vi "HandleObservationSync_002.vi"(8 "error in (no error)":errorcluster, 11 "S4GUI in":refnum<class "S4GUI.lvclass">) -> (0 "error out":errorcluster, 3 "S4GUI out":refnum<class "S4GUI.lvclass">)   [LabVIEW 2018, in "S4GUI.lvclass"] (continued)
            }
          }
          n1271 = call "Write AcquisitionB.vi"("error in (no error)"=w3487, "Acquisition.lvclass"=w3489, "S4ACS_GUI in"=w3488) -> ("error out"=w3483:errorcluster, "S4ACS_GUI out"=w3482:refnum<class "S4GUI.lvclass">)  [unwired: 7 in]
          n1272 = call-dynamic "Read AcquisitionC.vi"("error in (no error)"=w3483, "S4ACS_GUI in"=w3482) -> ("error out"=w3440:errorcluster, "Acquisition.lvclass"=w3442:refnum<class "Acquisition.lvclass">, "S4ACS_GUI out"=w3485:refnum<class "S4GUI.lvclass">)  [unwired: 7 in]
          n1273 = call-dynamic "Read enabled.vi"("error in (no error)"=w3440, "Server in"=w3442) -> ("error out"=w3439:errorcluster, "enabled"=w3432:bool, "Server out"=w3441:refnum<class "Acquisition.lvclass">)  [unwired: 7 in]
          n1274 = call "Read connection.vi"("error in (no error)"=w3439, "Server in"=w3441) -> ("error out"=w3469:errorcluster, "connection"=w3452:bool, "Server out"=w3470:refnum<class "Acquisition.lvclass">)  [unwired: 7 in]
          n1275 = And(x=w3452, y=w3432) -> (x .and. y?=w3454:bool)
          n1276 = case shown="True" w3454 {
            tunnel: [w3558 w3567] -> w3486
            tunnel: [w3559 w3566] -> w3484
            tunnel: w3470 -> [w3559 w3564]
            tunnel: w3469 -> [w3558 w3563]
            tunnel: [w3555 u32 0 ("New_State")] -> w3461
            tunnel: w3432 -> [w3554 _]
            frame False {
              n1277 = Select(t=u32 4, s=w3554, f=u32 0) -> (s? t:f=w3555:u32)
            }
            frame True {
              n1278 = call-dynamic "Read Channel.vi"("error in (no error)"=w3563, "Acquisition in"=w3564) -> ("error out"=w3571:errorcluster, "Channel.lvclass"=w3572:refnum<class "Channel.lvclass">, "Acquisition out"=w3565:refnum<class "Acquisition.lvclass">)  [unwired: 7 in]
              n1279 = call-dynamic "Read State Machine.vi"("error in (no error)"=w3571, "Device in"=w3572) -> ("error out"=w3570:errorcluster, "State Machine.lvclass"=w3568:refnum<class "State Machine.lvclass">, "Device out"=w3574:refnum<class "Channel.lvclass">)  [unwired: 7 in]
              n1280 = call "Next State.vi"("error in (no error)"=w3570, "New_State"=50, "State Machine in"=w3568) -> ("error out"=w3562:errorcluster, "State Machine out"=w3561:refnum<class "State Machine.lvclass">)  [unwired: 7 in]
              n1281 = call-dynamic "Write State Machine.vi"("error in (no error)"=w3562, "State Machine.lvclass"=w3561, "Device in"=w3574) -> ("error out"=w3575:errorcluster, "Device out"=w3573:refnum<class "Channel.lvclass">)  [unwired: 7 in]
              n1282 = call-dynamic "Write Channel.vi"("error in (no error)"=w3575, "Channel.lvclass"=w3573, "Acquisition in"=w3565) -> ("error out"=w3567:errorcluster, "Acquisition out"=w3566:refnum<class "Acquisition.lvclass">)  [unwired: 7 in]
            }
          }
          n1283 = call-dynamic "Write AcquisitionC.vi"("error in (no error)"=w3486, "Acquisition.lvclass"=w3484, "S4ACS_GUI in"=w3485) -> ("error out"=w3480:errorcluster, "S4ACS_GUI out"=w3479:refnum<class "S4GUI.lvclass">)  [unwired: 7 in]
          n1284 = call-dynamic "Read AcquisitionD.vi"("error in (no error)"=w3480, "S4ACS_GUI in"=w3479) -> ("error out"=w3436:errorcluster, "Acquisition.lvclass"=w3438:refnum<class "Acquisition.lvclass">, "S4ACS_GUI out"=w3478:refnum<class "S4GUI.lvclass">)  [unwired: 7 in]
          n1285 = call-dynamic "Read enabled.vi"("error in (no error)"=w3436, "Server in"=w3438) -> ("error out"=w3435:errorcluster, "enabled"=w3431:bool, "Server out"=w3437:refnum<class "Acquisition.lvclass">)  [unwired: 7 in]
          n1286 = call "Read connection.vi"("error in (no error)"=w3435, "Server in"=w3437) -> ("error out"=w3467:errorcluster, "connection"=w3451:bool, "Server out"=w3468:refnum<class "Acquisition.lvclass">)  [unwired: 7 in]
          n1287 = And(x=w3451, y=w3431) -> (x .and. y?=w3453:bool)
          n1288 = case shown="True" w3453 {
            tunnel: w3467 -> [w3536 w3553]
            tunnel: [w3536 w3552] -> w3481
            tunnel: w3468 -> [w3537 w3543]
            tunnel: [w3537 w3541] -> w3477
            tunnel: [w3533 u32 0 ("New_State")] -> w3460
            tunnel: w3431 -> [w3532 _]
            frame False {
              n1289 = Select(t=u32 8, s=w3532, f=u32 0) -> (s? t:f=w3533:u32)
            }
            frame True {
              n1290 = call-dynamic "Read Channel.vi"("error in (no error)"=w3553, "Acquisition in"=w3543) -> ("error out"=w3548:errorcluster, "Channel.lvclass"=w3547:refnum<class "Channel.lvclass">, "Acquisition out"=w3542:refnum<class "Acquisition.lvclass">)  [unwired: 7 in]
              n1291 = call-dynamic "Read State Machine.vi"("error in (no error)"=w3548, "Device in"=w3547) -> ("error out"=w3549:errorcluster, "State Machine.lvclass"=w3551:refnum<class "State Machine.lvclass">, "Device out"=w3545:refnum<class "Channel.lvclass">)  [unwired: 7 in]
              n1292 = call "Next State.vi"("error in (no error)"=w3549, "New_State"=50, "State Machine in"=w3551) -> ("error out"=w3539:errorcluster, "State Machine out"=w3540:refnum<class "State Machine.lvclass">)  [unwired: 7 in]
              n1293 = call-dynamic "Write State Machine.vi"("error in (no error)"=w3539, "State Machine.lvclass"=w3540, "Device in"=w3545) -> ("error out"=w3544:errorcluster, "Device out"=w3546:refnum<class "Channel.lvclass">)  [unwired: 7 in]
              n1294 = call-dynamic "Write Channel.vi"("error in (no error)"=w3544, "Channel.lvclass"=w3546, "Acquisition in"=w3542) -> ("error out"=w3552:errorcluster, "Acquisition out"=w3541:refnum<class "Acquisition.lvclass">)  [unwired: 7 in]
            }
          }
          n1295 = call-dynamic "Write AcquisitionD.vi"("error in (no error)"=w3481, "Acquisition.lvclass"=w3477, "S4ACS_GUI in"=w3478) -> ("error out"=w3476:errorcluster, "S4ACS_GUI out"=w3475:refnum<class "S4GUI.lvclass">)  [unwired: 7 in]
          n1296 = Compound Arithmetic op=ADD(w3463, w3462, w3461, w3460) -> (w3464:u32)
          n1297 = case shown="0, Default" w3464 {
            tunnel: w3459 -> [w3501 _ _ _ _ _ _ _ _ _ _ _ _ _ _ _]
            tunnel: [w3500 u32 1 ("Obs_state") u32 1 ("Obs_state") u32 1 ("Obs_state") u32 1 ("Obs_state") u32 1 ("Obs_state") u32 1 ("Obs_state") u32 1 ("Obs_state") u32 1 ("Obs_state") u32 1 ("Obs_state") u32 1 ("Obs_state") u32 1 ("Obs_state") u32 1 ("Obs_state") u32 1 ("Obs_state") u32 1 ("Obs_state") u32 1 ("Obs_state")] -> w3465
            tunnel: ["" ("Error Msg") "ERROR: Lost channel 1 connection... - HandleObservationSync.vi state 323" ("Error Msg") "ERROR: Lost channel 2 connection...- HandleObservationSync.vi state 323" ("Error Msg") "ERROR: Lost channels 1 and 2 connection...- HandleObservationSync.vi state 323" ("Error Msg") "ERROR: Lost channel 3 connection...- HandleObservationSync.vi state 323" ("Error Msg") "ERROR: Lost channels 1 and  3 connection...- HandleObservationSync.vi state 323" ("Error Msg") "ERROR:  Lost channels 2 and  3 connection...- HandleObservationSync.vi state 323" ("Error Msg") "ERROR:  Lost channels 1, 2 and  3 connection...- HandleObservationSync.vi state 323" ("Error Msg") "ERROR: Lost channel 4 connection...- HandleObservationSync.vi state 323" ("Error Msg") "ERROR:  Lost channels 1 and 4 connection...- HandleObservationSync.vi state 323" ("Error Msg") "ERROR:  Lost channels 2 and 4 connection...- HandleObservationSync.vi state 323" ("Error Msg") "ERROR: Lost channels 1, 2 and 4 connection...- HandleObservationSync.vi state 323" ("Error Msg") "ERROR: Lost channels 3 and 4 connection...- HandleObservationSync.vi state 323" ("Error Msg") "ERROR: Lost channels 1, 3 and 4 connection...- HandleObservationSync.vi state 323" ("Error Msg") "ERROR: Lost channels 2, 3 and 4 connection...- HandleObservationSync.vi state 323" ("Error Msg") "ERROR: Lost channels 1, 2, 3 and 4 connection...- HandleObservationSync.vi state 323" ("Error Msg")] -> w3466
            frame 0, Default {
              n1298 = Increment(x=w3501) -> (x+1=w3500:u32)
              n1299 = Tick Count (ms)() -> (millisecond timer value=w3498:u32)
              n1300 = local write "time1"(w3498) -> ()
            }
            frame 1 {
            }
            frame 2 {
            }
            frame 3 {
            }
            frame 4 {
            }
            frame 5 {
            }
            frame 6 {
            }
            frame 7 {
            }
            frame 8 {
            }
            frame 9 {
            }
            frame 10 {
            }
            frame 11 {
            }
            frame 12 {
            }
            frame 13 {
            }
            frame 14 {
            }
            frame 15 {
            }
          }
          n1301 = Bundle By Name(cluster=w3475, "Obs_state"=w3465, "Error Msg"=w3466) -> (w3492:refnum<class "S4GUI.lvclass">)
        }
        frame 324 {
          # "Espera terminar a execução do comando atual \nantes de ir ao proximo passo da Observação."
          n1302 = call-dynamic "Read AcquisitionA.vi"("error in (no error)"=w3670, "S4ACS_GUI in"=w3671) -> ("error out"=w3651:errorcluster, "Acquisition.lvclass"=w3652:refnum<class "Acquisition.lvclass">, "S4ACS_GUI out"=w3673:refnum<class "S4GUI.lvclass">)  [unwired: 7 in]
          n1303 = call "Read connection.vi"("error in (no error)"=w3651, "Server in"=w3652) -> ("error out"=w3650:errorcluster, "connection"=w3649:bool, "Server out"=w3648:refnum<class "Acquisition.lvclass">)  [unwired: 7 in]
          n1304 = case shown="True" w3649 {
            tunnel: w3650 -> [w3770 w3791]
            tunnel: [w3771 w3789] -> w3674
            tunnel: [w3770 w3788] -> w3672
            tunnel: [TRUE w3777] -> w3630
            tunnel: w3648 -> [w3771 w3780]
            tunnel: [FALSE w3772] -> w3628
            frame False {
            }
            frame True {
              n1305 = call-dynamic "Read Channel.vi"("error in (no error)"=w3791, "Acquisition in"=w3780) -> ("error out"=w3774:errorcluster, "Channel.lvclass"=w3776:refnum<class "Channel.lvclass">, "Acquisition out"=w3790:refnum<class "Acquisition.lvclass">)  [unwired: 7 in]
              n1306 = call-dynamic "Read wait_expose.vi"("error in (no error)"=w3774, "Channel in"=w3776) -> ("error out"=w3773:errorcluster, "wait_expose"=w3772:bool, "Channel out"=w3775:refnum<class "Channel.lvclass">)  [unwired: 7 in]
              n1307 = call-dynamic "Read State Machine.vi"("error in (no error)"=w3773, "Device in"=w3775) -> ("error out"=w3782:errorcluster, "State Machine.lvclass"=w3784:refnum<class "State Machine.lvclass">, "Device out"=w3786:refnum<class "Channel.lvclass">)  [unwired: 7 in]
              n1308 = call-dynamic "Read State.vi"("error in (no error)"=w3782, "State Machine in"=w3784) -> ("error out"=w3781:errorcluster, "State"=w3778:i32, "State Machine out"=w3783:refnum<class "State Machine.lvclass">)  [unwired: 7 in]
              n1309 = Greater?(x=w3778, y=53 ("x")) -> (0:w3777:bool)
              n1310 = call-dynamic "Write State Machine.vi"("error in (no error)"=w3781, "State Machine.lvclass"=w3783, "Device in"=w3786) -> ("error out"=w3785:errorcluster, "Device out"=w3787:refnum<class "Channel.lvclass">)  [unwired: 7 in]
              n1311 = call-dynamic "Write Channel.vi"("error in (no error)"=w3785, "Channel.lvclass"=w3787, "Acquisition in"=w3790) -> ("error out"=w3788:errorcluster, "Acquisition out"=w3789:refnum<class "Acquisition.lvclass">)  [unwired: 7 in]
            }
          }
          n1312 = call-dynamic "Write AcquisitionA.vi"("error in (no error)"=w3672, "Acquisition.lvclass"=w3674, "S4ACS_GUI in"=w3673) -> ("error out"=w3667:errorcluster, "S4ACS_GUI out"=w3666:refnum<class "S4GUI.lvclass">)  [unwired: 7 in]
          n1313 = call "Read AcquisitionB.vi"("error in (no error)"=w3667, "S4ACS_GUI in"=w3666) -> ("error out"=w3643:errorcluster, "Acquisition.lvclass"=w3647:refnum<class "Acquisition.lvclass">, "S4ACS_GUI out"=w3668:refnum<class "S4GUI.lvclass">)  [unwired: 7 in]
          n1314 = call "Read connection.vi"("error in (no error)"=w3643, "Server in"=w3647) -> ("error out"=w3644:errorcluster, "connection"=w3645:bool, "Server out"=w3646:refnum<class "Acquisition.lvclass">)  [unwired: 7 in]
          n1315 = case shown="True" w3645 {
            tunnel: w3644 -> [w3746 w3759]
            tunnel: w3646 -> [w3747 w3758]
            tunnel: [TRUE w3753] -> w3632
            tunnel: [w3746 w3757] -> w3665
            tunnel: [w3747 w3756] -> w3664
            tunnel: [FALSE w3748] -> w3627
            frame False {
            }
            frame True {
              n1316 = call-dynamic "Read Channel.vi"("error in (no error)"=w3759, "Acquisition in"=w3758) -> ("error out"=w3750:errorcluster, "Channel.lvclass"=w3752:refnum<class "Channel.lvclass">, "Acquisition out"=w3760:refnum<class "Acquisition.lvclass">)  [unwired: 7 in]
              n1317 = call-dynamic "Read wait_expose.vi"("error in (no error)"=w3750, "Channel in"=w3752) -> ("error out"=w3749:errorcluster, "wait_expose"=w3748:bool, "Channel out"=w3751:refnum<class "Channel.lvclass">)  [unwired: 7 in]
              n1318 = call-dynamic "Read State Machine.vi"("error in (no error)"=w3749, "Device in"=w3751) -> ("error out"=w3766:errorcluster, "State Machine.lvclass"=w3764:refnum<class "State Machine.lvclass">, "Device out"=w3762:refnum<class "Channel.lvclass">)  [unwired: 7 in]
              n1319 = call-dynamic "Read State.vi"("error in (no error)"=w3766, "State Machine in"=w3764) -> ("error out"=w3767:errorcluster, "State"=w3755:i32, "State Machine out"=w3765:refnum<class "State Machine.lvclass">)  [unwired: 7 in]
              n1320 = Greater?(x=w3755, y=53 ("x")) -> (0:w3753:bool)
              n1321 = call-dynamic "Write State Machine.vi"("error in (no error)"=w3767, "State Machine.lvclass"=w3765, "Device in"=w3762) -> ("error out"=w3763:errorcluster, "Device out"=w3761:refnum<class "Channel.lvclass">)  [unwired: 7 in]
              n1322 = call-dynamic "Write Channel.vi"("error in (no error)"=w3763, "Channel.lvclass"=w3761, "Acquisition in"=w3760) -> ("error out"=w3757:errorcluster, "Acquisition out"=w3756:refnum<class "Acquisition.lvclass">)  [unwired: 7 in]
            }
          }
          n1323 = call "Write AcquisitionB.vi"("error in (no error)"=w3665, "Acquisition.lvclass"=w3664, "S4ACS_GUI in"=w3668) -> ("error out"=w3657:errorcluster, "S4ACS_GUI out"=w3656:refnum<class "S4GUI.lvclass">)  [unwired: 7 in]
          n1324 = call-dynamic "Read AcquisitionC.vi"("error in (no error)"=w3657, "S4ACS_GUI in"=w3656) -> ("error out"=w3639:errorcluster, "Acquisition.lvclass"=w3642:refnum<class "Acquisition.lvclass">, "S4ACS_GUI out"=w3659:refnum<class "S4GUI.lvclass">)  [unwired: 7 in]
          n1325 = call "Read connection.vi"("error in (no error)"=w3639, "Server in"=w3642) -> ("error out"=w3638:errorcluster, "connection"=w3640:bool, "Server out"=w3641:refnum<class "Acquisition.lvclass">)  [unwired: 7 in]
          n1326 = case shown="True" w3640 {
            tunnel: [w3722 w3736] -> w3660
            tunnel: [w3723 w3735] -> w3658
            tunnel: w3638 -> [w3722 w3732]
            tunnel: w3641 -> [w3723 w3733]
            tunnel: [TRUE w3729] -> w3631
            tunnel: [FALSE w3724] -> w3626
            frame False {
            }
            frame True {
              n1327 = call-dynamic "Read Channel.vi"("error in (no error)"=w3732, "Acquisition in"=w3733) -> ("error out"=w3726:errorcluster, "Channel.lvclass"=w3728:refnum<class "Channel.lvclass">, "Acquisition out"=w3734:refnum<class "Acquisition.lvclass">)  [unwired: 7 in]
              n1328 = call-dynamic "Read wait_expose.vi"("error in (no error)"=w3726, "Channel in"=w3728) -> ("error out"=w3725:errorcluster, "wait_expose"=w3724:bool, "Channel out"=w3727:refnum<class "Channel.lvclass">)  [unwired: 7 in]
              n1329 = call-dynamic "Read State Machine.vi"("error in (no error)"=w3725, "Device in"=w3727) -> ("error out"=w3742:errorcluster, "State Machine.lvclass"=w3740:refnum<class "State Machine.lvclass">, "Device out"=w3738:refnum<class "Channel.lvclass">)  [unwired: 7 in]
              n1330 = call-dynamic "Read State.vi"("error in (no error)"=w3742, "State Machine in"=w3740) -> ("error out"=w3743:errorcluster, "State"=w3730:i32, "State Machine out"=w3741:refnum<class "State Machine.lvclass">)  [unwired: 7 in]
              n1331 = Greater?(x=w3730, y=53 ("x")) -> (0:w3729:bool)
              n1332 = call-dynamic "Write State Machine.vi"("error in (no error)"=w3743, "State Machine.lvclass"=w3741, "Device in"=w3738) -> ("error out"=w3739:errorcluster, "Device out"=w3737:refnum<class "Channel.lvclass">)  [unwired: 7 in]
              n1333 = call-dynamic "Write Channel.vi"("error in (no error)"=w3739, "Channel.lvclass"=w3737, "Acquisition in"=w3734) -> ("error out"=w3736:errorcluster, "Acquisition out"=w3735:refnum<class "Acquisition.lvclass">)  [unwired: 7 in]
            }
          }
          n1334 = call-dynamic "Write AcquisitionC.vi"("error in (no error)"=w3660, "Acquisition.lvclass"=w3658, "S4ACS_GUI in"=w3659) -> ("error out"=w3654:errorcluster, "S4ACS_GUI out"=w3655:refnum<class "S4GUI.lvclass">)  [unwired: 7 in]
          n1335 = call-dynamic "Read AcquisitionD.vi"("error in (no error)"=w3654, "S4ACS_GUI in"=w3655) -> ("error out"=w3634:errorcluster, "Acquisition.lvclass"=w3637:refnum<class "Acquisition.lvclass">, "S4ACS_GUI out"=w3661:refnum<class "S4GUI.lvclass">)  [unwired: 7 in]
          n1336 = call "Read connection.vi"("error in (no error)"=w3634, "Server in"=w3637) -> ("error out"=w3633:errorcluster, "connection"=w3635:bool, "Server out"=w3636:refnum<class "Acquisition.lvclass">)  [unwired: 7 in]
          n1337 = case shown="True" w3635 {
            tunnel: [w3699 w3719] -> w3663
            tunnel: [w3698 w3718] -> w3662
            tunnel: w3636 -> [w3699 w3717]
            tunnel: w3633 -> [w3698 w3716]
            tunnel: [TRUE w3705] -> w3629
            tunnel: [FALSE w3700] -> w3625
            frame False {
            }
            frame True {
              n1338 = call-dynamic "Read Channel.vi"("error in (no error)"=w3716, "Acquisition in"=w3717) -> ("error out"=w3702:errorcluster, "Channel.lvclass"=w3704:refnum<class "Channel.lvclass">, "Acquisition out"=w3715:refnum<class "Acquisition.lvclass">)  [unwired: 7 in]
              n1339 = call-dynamic "Read wait_expose.vi"("error in (no error)"=w3702, "Channel in"=w3704) -> ("error out"=w3701:errorcluster, "wait_expose"=w3700:bool, "Channel out"=w3703:refnum<class "Channel.lvclass">)  [unwired: 7 in]
              n1340 = call-dynamic "Read State Machine.vi"("error in (no error)"=w3701, "Device in"=w3703) -> ("error out"=w3709:errorcluster, "State Machine.lvclass"=w3711:refnum<class "State Machine.lvclass">, "Device out"=w3713:refnum<class "Channel.lvclass">)  [unwired: 7 in]
              n1341 = call-dynamic "Read State.vi"("error in (no error)"=w3709, "State Machine in"=w3711) -> ("error out"=w3708:errorcluster, "State"=w3706:i32, "State Machine out"=w3710:refnum<class "State Machine.lvclass">)  [unwired: 7 in]
              n1342 = Greater?(x=w3706, y=53 ("x")) -> (0:w3705:bool)
              n1343 = call-dynamic "Write State Machine.vi"("error in (no error)"=w3708, "State Machine.lvclass"=w3710, "Device in"=w3713) -> ("error out"=w3712:errorcluster, "Device out"=w3714:refnum<class "Channel.lvclass">)  [unwired: 7 in]
              n1344 = call-dynamic "Write Channel.vi"("error in (no error)"=w3712, "Channel.lvclass"=w3714, "Acquisition in"=w3715) -> ("error out"=w3718:errorcluster, "Acquisition out"=w3719:refnum<class "Acquisition.lvclass">)  [unwired: 7 in]
            }
          }
          n1345 = call-dynamic "Write AcquisitionD.vi"("error in (no error)"=w3662, "Acquisition.lvclass"=w3663, "S4ACS_GUI in"=w3661) -> ("error out"=w3653:errorcluster, "S4ACS_GUI out"=w3624:refnum<class "S4GUI.lvclass">)  [unwired: 7 in]
          n1346 = Compound Arithmetic op=AND(w3630, w3632, w3631, w3629) -> (w3623:bool)
          n1347 = Compound Arithmetic op=OR(w3628, w3627, w3626, w3625) -> (w3621:bool)
          n1348 = case shown="True" w3623 {
            tunnel: w3624 -> [w3676 w3695]
            tunnel: [w3682 w3694] -> w3620
            tunnel: w3622 -> [_ w3693]
            tunnel: w3621 -> [_ w3689]
            frame False {
              # "Aguardando iniciar exposição por 5s"
              n1349 = Tick Count (ms)() -> (millisecond timer value=w3681:u32)
              n1350 = local read "time1"() -> (w3675:u32)
              n1351 = Subtract(x=w3681, y=w3675) -> (x-y=w3678:u32)
              n1352 = To Double Precision Float(number=w3678) -> (double precision float=w3680:dbl)
              n1353 = Less?(x=5000.0 ("y"), y=w3680) -> (x < y?=w3679:bool)
              n1354 = case shown="True" w3679 {
                tunnel: w3676 -> [w3683 w3687]
                tunnel: [w3683 w3686] -> w3682
                frame False {
                }
                frame True {
                  n1355 = Bundle By Name(cluster=w3687, "Obs_state"=u32 1, "Error Msg"="ERROR: Acquisition Timeout. HandleObservationSync.vi - state 324.") -> (w3686:refnum<class "S4GUI.lvclass">)
                }
              }
            }
            frame True {
              # "327: Verifica incremento de ciclo."
              # "Iniciou aquisição..."
              n1356 = Increment(x=w3693) -> (x+1=w3690:u32)
              n1357 = Select(t=u32 327, s=w3689, f=w3690) -> (s? t:f=w3688:u32)
              n1358 = Tick Count (ms)() -> (millisecond timer value=w3692:u32)
              n1359 = Bundle By Name(cluster=w3695, "Obs_state"=w3688) -> (w3694:refnum<class "S4GUI.lvclass">)
              n1360 = local write "time307"(w3692) -> ()
            }
          }
          n1361 = Bundle By Name(cluster=w3620, "mode EXPOSE"=w3621) -> (w3669:refnum<class "S4GUI.lvclass">)
        }
        frame 325 {
          n1362 = Unbundle By Name(w3801) -> ("mode EXPOSE"=w3800:bool)
          n1363 = case shown="True" w3800 {
            tunnel: w3801 -> [w3854 w3921]
            tunnel: w3806 -> [w3853 w3920]
            tunnel: [w3852 w3918] -> w3805
            tunnel: [w3851 w3919] -> w3804
            tunnel: [w3850 w3917] -> w3794
            tunnel: w3802 -> [w3842 w3917]
            tunnel: [w3841 w3882] -> w3799
            tunnel: [w3841 w3881] -> w3798
            tunnel: [w3841 w3880] -> w3797
            tunnel: [w3841 w3879] -> w3796
            frame False {
              w3841 = 0
              n1364 = call-dynamic "Read Sync Box.lvclass.vi"("error in (no error)"=w3853, "SPARC4_AC in"=w3854) -> ("error out"=w3847:errorcluster, "Sync Box.lvclass"=w3849:refnum<class "Sync Box.lvclass">, "SPARC4_AC out"=w3844:refnum<class "S4GUI.lvclass">)  [unwired: 7 in]
              n1365 = call "Read connection.vi"("error in (no error)"=w3847, "Server in"=w3849) -> ("error out"=w3846:errorcluster, "connection"=w3845:bool, "Server out"=w3848:refnum<class "Sync Box.lvclass">)  [unwired: 7 in]
              n1366 = case shown="True" w3845 {
                tunnel: w3846 -> [w3860 w3878]
                tunnel: [w3861 w3876] -> w3856
                tunnel: [w3860 w3863] -> w3855
                tunnel: w3842 -> [w3857 w3862]
                tunnel: [w3859 w3862] -> w3850
                tunnel: w3848 -> [w3861 w3867]
                tunnel: w3844 -> [w3858 w3864]
                tunnel: [w3858 w3864] -> w3843
                frame False {
                  n1367 = Increment(x=w3857) -> (x+1=w3859:u32)
                }
                frame True {
                  # "Envia comando FIRE para o SyncBox"
                  n1368 = call-dynamic "Read Trigger.lvclass.vi"("error in (no error)"=w3878, "Sync Box in"=w3867) -> ("error out"=w3872:errorcluster, "Trigger.lvclass"=w3871:refnum<class "Trigger.lvclass">, "Sync Box out"=w3877:refnum<class "Sync Box.lvclass">)  [unwired: 7 in]
                  n1369 = call-dynamic "Read State Machine.vi"("error in (no error)"=w3872, "Device in"=w3871) -> ("error out"=w3873:errorcluster, "State Machine.lvclass"=w3875:refnum<class "State Machine.lvclass">, "Device out"=w3869:refnum<class "Trigger.lvclass">)  [unwired: 7 in]
                  n1370 = call "Next State.vi"("error in (no error)"=w3873, "New_State"=40, "State Machine in"=w3875) -> ("error out"=w3865:errorcluster, "State Machine out"=w3866:refnum<class "State Machine.lvclass">)  [unwired: 7 in]
                  n1371 = call-dynamic "Write State Machine.vi"("error in (no error)"=w3865, "State Machine.lvclass"=w3866, "Device in"=w3869) -> ("error out"=w3868:errorcluster, "Device out"=w3870:refnum<class "Trigger.lvclass">)  [unwired: 7 in]
                  n1372 = call-dynamic "Write Trigger.lvclass.vi"("error in (no error)"=w3868, "Trigger.lvclass"=w3870, "Sync Box in"=w3877) -> ("error out"=w3863:errorcluster, "Sync Box out"=w3876:refnum<class "Sync Box.lvclass">)  [unwired: 7 in]
                }
              }
              n1373 = call-dynamic "Write Sync Box.lvclass.vi"("error in (no error)"=w3855, "Sync Box.lvclass"=w3856, "SPARC4_AC in"=w3843) -> ("error out"=w3852:errorcluster, "SPARC4_AC out"=w3851:refnum<class "S4GUI.lvclass">)  [unwired: 7 in]
            }
            frame True {
              # "Envia comando EXPOSE para os canais ativos"
              n1374 = call-dynamic "Read AcquisitionA.vi"("error in (no error)"=w3920, "S4ACS_GUI in"=w3921) -> ("error out"=w3914:errorcluster, "Acquisition.lvclass"=w3916:refnum<class "Acquisition.lvclass">, "S4ACS_GUI out"=w3940:refnum<class "S4GUI.lvclass">)  [unwired: 7 in]
              n1375 = call-dynamic "Read enabled.vi"("error in (no error)"=w3914, "Server in"=w3916) -> ("error out"=w3913:errorcluster, "enabled"=w3886:bool, "Server out"=w3915:refnum<class "Acquisition.lvclass">)  [unwired: 7 in]
              n1376 = call "Read connection.vi"("error in (no error)"=w3913, "Server in"=w3915) -> ("error out"=w3922:errorcluster, "connection"=w3911:bool, "Server out"=w3923:refnum<class "Acquisition.lvclass">)  [unwired: 7 in]
              n1377 = And(x=w3911, y=w3886) -> (x .and. y?=w3912:bool)
              n1378 = case shown="True" w3912 {
                tunnel: w3923 -> [w4013 w4029]
                tunnel: w3922 -> [w4012 w4028]
                tunnel: [w4013 w4026] -> w3941
                tunnel: [w4012 w4025] -> w3939
                tunnel: [w4008 0] -> w3882
                tunnel: w3886 -> [w4009 _]
                frame False {
                  n1379 = Select(t=1, s=w4009, f=0) -> (s? t:f=w4008:i32)
                }
                frame True {
                  n1380 = call-dynamic "Read Channel.vi"("error in (no error)"=w4028, "Acquisition in"=w4029) -> ("error out"=w4021:errorcluster, "Channel.lvclass"=w4020:refnum<class "Channel.lvclass">, "Acquisition out"=w4027:refnum<class "Acquisition.lvclass">)  [unwired: 7 in]
                  n1381 = call-dynamic "Read State Machine.vi"("error in (no error)"=w4021, "Device in"=w4020) -> ("error out"=w4022:errorcluster, "State Machine.lvclass"=w4024:refnum<class "State Machine.lvclass">, "Device out"=w4018:refnum<class "Channel.lvclass">)  [unwired: 7 in]
                  n1382 = call "Next State.vi"("error in (no error)"=w4022, "New_State"=50, "State Machine in"=w4024) -> ("error out"=w4015:errorcluster, "State Machine out"=w4016:refnum<class "State Machine.lvclass">)  [unwired: 7 in]
                  n1383 = call-dynamic "Write State Machine.vi"("error in (no error)"=w4015, "State Machine.lvclass"=w4016, "Device in"=w4018) -> ("error out"=w4017:errorcluster, "Device out"=w4019:refnum<class "Channel.lvclass">)  [unwired: 7 in]
                  n1384 = call-dynamic "Write Channel.vi"("error in (no error)"=w4017, "Channel.lvclass"=w4019, "Acquisition in"=w4027) -> ("error out"=w4025:errorcluster, "Acquisition out"=w4026:refnum<class "Acquisition.lvclass">)  [unwired: 7 in]
                }
              }
              n1385 = call-dynamic "Write AcquisitionA.vi"("error in (no error)"=w3939, "Acquisition.lvclass"=w3941, "S4ACS_GUI in"=w3940) -> ("error out"=w3937:errorcluster, "S4ACS_GUI out"=w3938:refnum<class "S4GUI.lvclass">)  [unwired: 7 in]
              n1386 = call "Read AcquisitionB.vi"("error in (no error)"=w3937, "S4ACS_GUI in"=w3938) -> ("error out"=w3905:errorcluster, "Acquisition.lvclass"=w3907:refnum<class "Acquisition.lvclass">, "S4ACS_GUI out"=w3935:refnum<class "S4GUI.lvclass">)  [unwired: 7 in]
              n1387 = call-dynamic "Read enabled.vi"("error in (no error)"=w3905, "Server in"=w3907) -> ("error out"=w3909:errorcluster, "enabled"=w3885:bool, "Server out"=w3910:refnum<class "Acquisition.lvclass">)  [unwired: 7 in]
              n1388 = call "Read connection.vi"("error in (no error)"=w3909, "Server in"=w3910) -> ("error out"=w3904:errorcluster, "connection"=w3908:bool, "Server out"=w3906:refnum<class "Acquisition.lvclass">)  [unwired: 7 in]
              n1389 = And(x=w3908, y=w3885) -> (x .and. y?=w3903:bool)
              n1390 = case shown="False" w3903 {
                tunnel: w3906 -> [w3991 w4007]
                tunnel: w3904 -> [w3990 w4006]
                tunnel: [w3991 w4004] -> w3936
                tunnel: [w3990 w4003] -> w3934
                tunnel: [w3987 0] -> w3881
                tunnel: w3885 -> [w3986 _]
                frame False {
                  n1391 = Select(t=2, s=w3986, f=0) -> (s? t:f=w3987:i32)
                }
                frame True {
                  n1392 = call-dynamic "Read Channel.vi"("error in (no error)"=w4006, "Acquisition in"=w4007) -> ("error out"=w3999:errorcluster, "Channel.lvclass"=w3998:refnum<class "Channel.lvclass">, "Acquisition out"=w4005:refnum<class "Acquisition.lvclass">)  [unwired: 7 in]
                  n1393 = call-dynamic "Read State Machine.vi"("error in (no error)"=w3999, "Device in"=w3998) -> ("error out"=w4000:errorcluster, "State Machine.lvclass"=w4002:refnum<class "State Machine.lvclass">, "Device out"=w3996:refnum<class "Channel.lvclass">)  [unwired: 7 in]
                  n1394 = call "Next State.vi"("error in (no error)"=w4000, "New_State"=50, "State Machine in"=w4002) -> ("error out"=w3993:errorcluster, "State Machine out"=w3994:refnum<class "State Machine.lvclass">)  [unwired: 7 in]
                  n1395 = call-dynamic "Write State Machine.vi"("error in (no error)"=w3993, "State Machine.lvclass"=w3994, "Device in"=w3996) -> ("error out"=w3995:errorcluster, "Device out"=w3997:refnum<class "Channel.lvclass">)  [unwired: 7 in]
                  n1396 = call-dynamic "Write Channel.vi"("error in (no error)"=w3995, "Channel.lvclass"=w3997, "Acquisition in"=w4005) -> ("error out"=w4003:errorcluster, "Acquisition out"=w4004:refnum<class "Acquisition.lvclass">)  [unwired: 7 in]
                }
              }
              n1397 = call "Write AcquisitionB.vi"("error in (no error)"=w3934, "Acquisition.lvclass"=w3936, "S4ACS_GUI in"=w3935) -> ("error out"=w3930:errorcluster, "S4ACS_GUI out"=w3929:refnum<class "S4GUI.lvclass">)  [unwired: 7 in]
              n1398 = call-dynamic "Read AcquisitionC.vi"("error in (no error)"=w3930, "S4ACS_GUI in"=w3929) -> ("error out"=w3896:errorcluster, "Acquisition.lvclass"=w3897:refnum<class "Acquisition.lvclass">, "S4ACS_GUI out"=w3932:refnum<class "S4GUI.lvclass">)  [unwired: 7 in]
              n1399 = call-dynamic "Read enabled.vi"("error in (no error)"=w3896, "Server in"=w3897) -> ("error out"=w3901:errorcluster, "enabled"=w3884:bool, "Server out"=w3902:refnum<class "Acquisition.lvclass">)  [unwired: 7 in]
              n1400 = call "Read connection.vi"("error in (no error)"=w3901, "Server in"=w3902) -> ("error out"=w3898:errorcluster, "connection"=w3900:bool, "Server out"=w3899:refnum<class "Acquisition.lvclass">)  [unwired: 7 in]
              n1401 = And(x=w3900, y=w3884) -> (x .and. y?=w3895:bool)
              n1402 = case shown="False" w3895 {
                tunnel: [w3968 w3977] -> w3933
                tunnel: [w3969 w3976] -> w3931
                tunnel: w3899 -> [w3969 w3974]
                tunnel: w3898 -> [w3968 w3973]
                tunnel: [w3964 0] -> w3880
                tunnel: w3884 -> [w3965 _]
                frame False {
                  n1403 = Select(t=4, s=w3965, f=0) -> (s? t:f=w3964:i32)
                }
                frame True {
                  n1404 = call-dynamic "Read Channel.vi"("error in (no error)"=w3973, "Acquisition in"=w3974) -> ("error out"=w3981:errorcluster, "Channel.lvclass"=w3982:refnum<class "Channel.lvclass">, "Acquisition out"=w3975:refnum<class "Acquisition.lvclass">)  [unwired: 7 in]
                  n1405 = call-dynamic "Read State Machine.vi"("error in (no error)"=w3981, "Device in"=w3982) -> ("error out"=w3980:errorcluster, "State Machine.lvclass"=w3978:refnum<class "State Machine.lvclass">, "Device out"=w3984:refnum<class "Channel.lvclass">)  [unwired: 7 in]
                  n1406 = call "Next State.vi"("error in (no error)"=w3980, "New_State"=50, "State Machine in"=w3978) -> ("error out"=w3972:errorcluster, "State Machine out"=w3971:refnum<class "State Machine.lvclass">)  [unwired: 7 in]
                  n1407 = call-dynamic "Write State Machine.vi"("error in (no error)"=w3972, "State Machine.lvclass"=w3971, "Device in"=w3984) -> ("error out"=w3985:errorcluster, "Device out"=w3983:refnum<class "Channel.lvclass">)  [unwired: 7 in]
                  n1408 = call-dynamic "Write Channel.vi"("error in (no error)"=w3985, "Channel.lvclass"=w3983, "Acquisition in"=w3975) -> ("error out"=w3977:errorcluster, "Acquisition out"=w3976:refnum<class "Acquisition.lvclass">)  [unwired: 7 in]
                }
              }
              n1409 = call-dynamic "Write AcquisitionC.vi"("error in (no error)"=w3933, "Acquisition.lvclass"=w3931, "S4ACS_GUI in"=w3932) -> ("error out"=w3927:errorcluster, "S4ACS_GUI out"=w3926:refnum<class "S4GUI.lvclass">)  [unwired: 7 in]
              n1410 = call-dynamic "Read AcquisitionD.vi"("error in (no error)"=w3927, "S4ACS_GUI in"=w3926) -> ("error out"=w3888:errorcluster, "Acquisition.lvclass"=w3889:refnum<class "Acquisition.lvclass">, "S4ACS_GUI out"=w3925:refnum<class "S4GUI.lvclass">)  [unwired: 7 in]
              n1411 = call-dynamic "Read enabled.vi"("error in (no error)"=w3888, "Server in"=w3889) -> ("error out"=w3893:errorcluster, "enabled"=w3883:bool, "Server out"=w3894:refnum<class "Acquisition.lvclass">)  [unwired: 7 in]
              n1412 = call "Read connection.vi"("error in (no error)"=w3893, "Server in"=w3894) -> ("error out"=w3891:errorcluster, "connection"=w3892:bool, "Server out"=w3890:refnum<class "Acquisition.lvclass">)  [unwired: 7 in]
              n1413 = And(x=w3892, y=w3883) -> (x .and. y?=w3887:bool)
              n1414 = case shown="False" w3887 {
                tunnel: w3891 -> [w3946 w3963]
                tunnel: [w3946 w3962] -> w3928
                tunnel: w3890 -> [w3947 w3953]
                tunnel: [w3947 w3951] -> w3924
                tunnel: [w3942 0] -> w3879
                tunnel: w3883 -> [w3943 _]
                frame False {
                  n1415 = Select(t=8, s=w3943, f=0) -> (s? t:f=w3942:i32)
                }
                frame True {
                  n1416 = call-dynamic "Read Channel.vi"("error in (no error)"=w3963, "Acquisition in"=w3953) -> ("error out"=w3958:errorcluster, "Channel.lvclass"=w3957:refnum<class "Channel.lvclass">, "Acquisition out"=w3952:refnum<class "Acquisition.lvclass">)  [unwired: 7 in]
                  n1417 = call-dynamic "Read State Machine.vi"("error in (no error)"=w3958, "Device in"=w3957) -> ("error out"=w3959:errorcluster, "State Machine.lvclass"=w3961:refnum<class "State Machine.lvclass">, "Device out"=w3955:refnum<class "Channel.lvclass">)  [unwired: 7 in]
                  n1418 = call "Next State.vi"("error in (no error)"=w3959, "New_State"=50, "State Machine in"=w3961) -> ("error out"=w3949:errorcluster, "State Machine out"=w3950:refnum<class "State Machine.lvclass">)  [unwired: 7 in]
                  n1419 = call-dynamic "Write State Machine.vi"("error in (no error)"=w3949, "State Machine.lvclass"=w3950, "Device in"=w3955) -> ("error out"=w3954:errorcluster, "Device out"=w3956:refnum<class "Channel.lvclass">)  [unwired: 7 in]
                  n1420 = call-dynamic "Write Channel.vi"("error in (no error)"=w3954, "Channel.lvclass"=w3956, "Acquisition in"=w3952) -> ("error out"=w3962:errorcluster, "Acquisition out"=w3951:refnum<class "Acquisition.lvclass">)  [unwired: 7 in]
                }
              }
              n1421 = call-dynamic "Write AcquisitionD.vi"("error in (no error)"=w3928, "Acquisition.lvclass"=w3924, "S4ACS_GUI in"=w3925) -> ("error out"=w3918:errorcluster, "S4ACS_GUI out"=w3919:refnum<class "S4GUI.lvclass">)  [unwired: 7 in]
            }
          }
          n1422 = Compound Arithmetic op=ADD(w3799, w3798, w3797, w3796) -> (w3795:i32)
          n1423 = case shown="0, Default" w3795 {
            tunnel: w3794 -> [w3810 _ _ _ _ _ _ _ _ _ _ _ _ _ _ _]
            tunnel: [w3809 u32 1 ("Obs_state") u32 1 ("Obs_state") u32 1 ("Obs_state") u32 1 ("Obs_state") u32 1 ("Obs_state") u32 1 ("Obs_state") u32 1 ("Obs_state") u32 1 ("Obs_state") u32 1 ("Obs_state") u32 1 ("Obs_state") u32 1 ("Obs_state") u32 1 ("Obs_state") u32 1 ("Obs_state") u32 1 ("Obs_state") u32 1 ("Obs_state")] -> w3793
            tunnel: ["" ("Error Msg") "ERROR: Lost channel 1 connection... - HandleObservationSync.vi state 325" ("Error Msg") "ERROR: Lost channel 2 connection...- HandleObservationSync.vi state 325" ("Error Msg") "ERROR: Lost channels 1 and 2 connection...- HandleObservationSync.vi state 325" ("Error Msg") "ERROR: Lost channel 3 connection...- HandleObservationSync.vi state 325" ("Error Msg") "ERROR: Lost channels 1 and  3 connection...- HandleObservationSync.vi state 325" ("Error Msg") "ERROR:  Lost channels 2 and  3 connection...- HandleObservationSync.vi state 325" ("Error Msg") "ERROR:  Lost channels 1, 2 and  3 connection...- HandleObservationSync.vi state 325" ("Error Msg") "ERROR: Lost channel 4 connection...- HandleObservationSync.vi state 325" ("Error Msg") "ERROR:  Lost channels 1 and 4 connection...- HandleObservationSync.vi state 325" ("Error Msg") "ERROR:  Lost channels 2 and 4 connection...- HandleObservationSync.vi state 325" ("Error Msg") "ERROR: Lost channels 1, 2 and 4 connection...- HandleObservationSync.vi state 325" ("Error Msg") "ERROR: Lost channels 3 and 4 connection...- HandleObservationSync.vi state 325" ("Error Msg") "ERROR: Lost channels 1, 3 and 4 connection...- HandleObservationSync.vi state 325" ("Error Msg") "ERROR: Lost channels 2, 3 and 4 connection...- HandleObservationSync.vi state 325" ("Error Msg") "ERROR: Lost channels 1, 2, 3 and 4 connection...- HandleObservationSync.vi state 325" ("Error Msg")] -> w3792
            frame 0, Default {
              n1424 = Increment(x=w3810) -> (x+1=w3809:u32)
              n1425 = Tick Count (ms)() -> (millisecond timer value=w3807:u32)
              n1426 = local write "time1"(w3807) -> ()
            }
            frame 1 {
            }
            frame 2 {
            }
            frame 3 {
            }
            frame 4 {
            }
            frame 5 {
            }
            frame 6 {
            }
            frame 7 {
            }
            frame 8 {
            }
            frame 9 {
            }
            frame 10 {
            }
            frame 11 {
            }
            frame 12 {
            }
            frame 13 {
            }
            frame 14 {
            }
            frame 15 {
            }
          }
          n1427 = Bundle By Name(cluster=w3804, "Obs_state"=w3793, "Error Msg"=w3792) -> (w3803:refnum<class "S4GUI.lvclass">)
        }
        frame 326 {
          # "Espera terminar a execução do comando atual \nantes de ir ao proximo passo da Observação."
          n1428 = call-dynamic "Read AcquisitionA.vi"("error in (no error)"=w4080, "S4ACS_GUI in"=w4081) -> ("error out"=w4061:errorcluster, "Acquisition.lvclass"=w4062:refnum<class "Acquisition.lvclass">, "S4ACS_GUI out"=w4083:refnum<class "S4GUI.lvclass">)  [unwired: 7 in]
          n1429 = call "Read connection.vi"("error in (no error)"=w4061, "Server in"=w4062) -> ("error out"=w4060:errorcluster, "connection"=w4059:bool, "Server out"=w4058:refnum<class "Acquisition.lvclass">)  [unwired: 7 in]
          n1430 = case shown="True" w4059 {
            tunnel: w4060 -> [w4167 w4188]
            tunnel: [w4168 w4186] -> w4084
            tunnel: [w4167 w4185] -> w4082
            tunnel: [TRUE w4174] -> w4040
            tunnel: w4058 -> [w4168 w4177]
            tunnel: [FALSE w4169] -> w4038
            frame False {
            }
            frame True {
              n1431 = call-dynamic "Read Channel.vi"("error in (no error)"=w4188, "Acquisition in"=w4177) -> ("error out"=w4171:errorcluster, "Channel.lvclass"=w4173:refnum<class "Channel.lvclass">, "Acquisition out"=w4187:refnum<class "Acquisition.lvclass">)  [unwired: 7 in]
              n1432 = call-dynamic "Read wait_expose.vi"("error in (no error)"=w4171, "Channel in"=w4173) -> ("error out"=w4170:errorcluster, "wait_expose"=w4169:bool, "Channel out"=w4172:refnum<class "Channel.lvclass">)  [unwired: 7 in]
              n1433 = call-dynamic "Read State Machine.vi"("error in (no error)"=w4170, "Device in"=w4172) -> ("error out"=w4179:errorcluster, "State Machine.lvclass"=w4181:refnum<class "State Machine.lvclass">, "Device out"=w4183:refnum<class "Channel.lvclass">)  [unwired: 7 in]
              n1434 = call-dynamic "Read State.vi"("error in (no error)"=w4179, "State Machine in"=w4181) -> ("error out"=w4178:errorcluster, "State"=w4175:i32, "State Machine out"=w4180:refnum<class "State Machine.lvclass">)  [unwired: 7 in]
              n1435 = Greater?(x=w4175, y=53 ("x")) -> (0:w4174:bool)
              n1436 = call-dynamic "Write State Machine.vi"("error in (no error)"=w4178, "State Machine.lvclass"=w4180, "Device in"=w4183) -> ("error out"=w4182:errorcluster, "Device out"=w4184:refnum<class "Channel.lvclass">)  [unwired: 7 in]
              n1437 = call-dynamic "Write Channel.vi"("error in (no error)"=w4182, "Channel.lvclass"=w4184, "Acquisition in"=w4187) -> ("error out"=w4185:errorcluster, "Acquisition out"=w4186:refnum<class "Acquisition.lvclass">)  [unwired: 7 in]
            }
          }
          n1438 = call-dynamic "Write AcquisitionA.vi"("error in (no error)"=w4082, "Acquisition.lvclass"=w4084, "S4ACS_GUI in"=w4083) -> ("error out"=w4077:errorcluster, "S4ACS_GUI out"=w4076:refnum<class "S4GUI.lvclass">)  [unwired: 7 in]
          n1439 = call "Read AcquisitionB.vi"("error in (no error)"=w4077, "S4ACS_GUI in"=w4076) -> ("error out"=w4053:errorcluster, "Acquisition.lvclass"=w4057:refnum<class "Acquisition.lvclass">, "S4ACS_GUI out"=w4078:refnum<class "S4GUI.lvclass">)  [unwired: 7 in]
          n1440 = call "Read connection.vi"("error in (no error)"=w4053, "Server in"=w4057) -> ("error out"=w4054:errorcluster, "connection"=w4055:bool, "Server out"=w4056:refnum<class "Acquisition.lvclass">)  [unwired: 7 in]
          n1441 = case shown="True" w4055 {
            tunnel: w4054 -> [w4143 w4156]
            tunnel: w4056 -> [w4144 w4155]
            tunnel: [TRUE w4150] -> w4042
            tunnel: [w4143 w4154] -> w4075
            tunnel: [w4144 w4153] -> w4074
            tunnel: [FALSE w4145] -> w4037
            frame False {
            }
            frame True {
              n1442 = call-dynamic "Read Channel.vi"("error in (no error)"=w4156, "Acquisition in"=w4155) -> ("error out"=w4147:errorcluster, "Channel.lvclass"=w4149:refnum<class "Channel.lvclass">, "Acquisition out"=w4157:refnum<class "Acquisition.lvclass">)  [unwired: 7 in]
              n1443 = call-dynamic "Read wait_expose.vi"("error in (no error)"=w4147, "Channel in"=w4149) -> ("error out"=w4146:errorcluster, "wait_expose"=w4145:bool, "Channel out"=w4148:refnum<class "Channel.lvclass">)  [unwired: 7 in]
              n1444 = call-dynamic "Read State Machine.vi"("error in (no error)"=w4146, "Device in"=w4148) -> ("error out"=w4163:errorcluster, "State Machine.lvclass"=w4161:refnum<class "State Machine.lvclass">, "Device out"=w4159:refnum<class "Channel.lvclass">)  [unwired: 7 in]
              n1445 = call-dynamic "Read State.vi"("error in (no error)"=w4163, "State Machine in"=w4161) -> ("error out"=w4164:errorcluster, "State"=w4152:i32, "State Machine out"=w4162:refnum<class "State Machine.lvclass">)  [unwired: 7 in]
              n1446 = Greater?(x=w4152, y=53 ("x")) -> (0:w4150:bool)
              n1447 = call-dynamic "Write State Machine.vi"("error in (no error)"=w4164, "State Machine.lvclass"=w4162, "Device in"=w4159) -> ("error out"=w4160:errorcluster, "Device out"=w4158:refnum<class "Channel.lvclass">)  [unwired: 7 in]
              n1448 = call-dynamic "Write Channel.vi"("error in (no error)"=w4160, "Channel.lvclass"=w4158, "Acquisition in"=w4157) -> ("error out"=w4154:errorcluster, "Acquisition out"=w4153:refnum<class "Acquisition.lvclass">)  [unwired: 7 in]
            }
          }
          n1449 = call "Write AcquisitionB.vi"("error in (no error)"=w4075, "Acquisition.lvclass"=w4074, "S4ACS_GUI in"=w4078) -> ("error out"=w4067:errorcluster, "S4ACS_GUI out"=w4066:refnum<class "S4GUI.lvclass">)  [unwired: 7 in]
          n1450 = call-dynamic "Read AcquisitionC.vi"("error in (no error)"=w4067, "S4ACS_GUI in"=w4066) -> ("error out"=w4049:errorcluster, "Acquisition.lvclass"=w4052:refnum<class "Acquisition.lvclass">, "S4ACS_GUI out"=w4069:refnum<class "S4GUI.lvclass">)  [unwired: 7 in]
          n1451 = call "Read connection.vi"("error in (no error)"=w4049, "Server in"=w4052) -> ("error out"=w4048:errorcluster, "connection"=w4050:bool, "Server out"=w4051:refnum<class "Acquisition.lvclass">)  [unwired: 7 in]
          n1452 = case shown="True" w4050 {
            tunnel: [w4119 w4133] -> w4070
            tunnel: [w4120 w4132] -> w4068
            tunnel: w4048 -> [w4119 w4129]
            tunnel: w4051 -> [w4120 w4130]
            tunnel: [TRUE w4126] -> w4041
            tunnel: [FALSE w4121] -> w4036
            frame False {
            }
            frame True {
              n1453 = call-dynamic "Read Channel.vi"("error in (no error)"=w4129, "Acquisition in"=w4130) -> ("error out"=w4123:errorcluster, "Channel.lvclass"=w4125:refnum<class "Channel.lvclass">, "Acquisition out"=w4131:refnum<class "Acquisition.lvclass">)  [unwired: 7 in]
              n1454 = call-dynamic "Read wait_expose.vi"("error in (no error)"=w4123, "Channel in"=w4125) -> ("error out"=w4122:errorcluster, "wait_expose"=w4121:bool, "Channel out"=w4124:refnum<class "Channel.lvclass">)  [unwired: 7 in]
              n1455 = call-dynamic "Read State Machine.vi"("error in (no error)"=w4122, "Device in"=w4124) -> ("error out"=w4139:errorcluster, "State Machine.lvclass"=w4137:refnum<class "State Machine.lvclass">, "Device out"=w4135:refnum<class "Channel.lvclass">)  [unwired: 7 in]
              n1456 = call-dynamic "Read State.vi"("error in (no error)"=w4139, "State Machine in"=w4137) -> ("error out"=w4140:errorcluster, "State"=w4127:i32, "State Machine out"=w4138:refnum<class "State Machine.lvclass">)  [unwired: 7 in]
              n1457 = Greater?(x=w4127, y=53 ("x")) -> (0:w4126:bool)
              n1458 = call-dynamic "Write State Machine.vi"("error in (no error)"=w4140, "State Machine.lvclass"=w4138, "Device in"=w4135) -> ("error out"=w4136:errorcluster, "Device out"=w4134:refnum<class "Channel.lvclass">)  [unwired: 7 in]
              n1459 = call-dynamic "Write Channel.vi"("error in (no error)"=w4136, "Channel.lvclass"=w4134, "Acquisition in"=w4131) -> ("error out"=w4133:errorcluster, "Acquisition out"=w4132:refnum<class "Acquisition.lvclass">)  [unwired: 7 in]
            }
          }
          n1460 = call-dynamic "Write AcquisitionC.vi"("error in (no error)"=w4070, "Acquisition.lvclass"=w4068, "S4ACS_GUI in"=w4069) -> ("error out"=w4064:errorcluster, "S4ACS_GUI out"=w4065:refnum<class "S4GUI.lvclass">)  [unwired: 7 in]
          n1461 = call-dynamic "Read AcquisitionD.vi"("error in (no error)"=w4064, "S4ACS_GUI in"=w4065) -> ("error out"=w4044:errorcluster, "Acquisition.lvclass"=w4047:refnum<class "Acquisition.lvclass">, "S4ACS_GUI out"=w4071:refnum<class "S4GUI.lvclass">)  [unwired: 7 in]
          n1462 = call "Read connection.vi"("error in (no error)"=w4044, "Server in"=w4047) -> ("error out"=w4043:errorcluster, "connection"=w4045:bool, "Server out"=w4046:refnum<class "Acquisition.lvclass">)  [unwired: 7 in]
          n1463 = case shown="True" w4045 {
            tunnel: [w4096 w4116] -> w4073
            tunnel: [w4095 w4115] -> w4072
            tunnel: w4046 -> [w4096 w4114]
            tunnel: w4043 -> [w4095 w4113]
            tunnel: [TRUE w4102] -> w4039
            tunnel: [FALSE w4097] -> w4035
            frame False {
            }
            frame True {
              n1464 = call-dynamic "Read Channel.vi"("error in (no error)"=w4113, "Acquisition in"=w4114) -> ("error out"=w4099:errorcluster, "Channel.lvclass"=w4101:refnum<class "Channel.lvclass">, "Acquisition out"=w4112:refnum<class "Acquisition.lvclass">)  [unwired: 7 in]
              n1465 = call-dynamic "Read wait_expose.vi"("error in (no error)"=w4099, "Channel in"=w4101) -> ("error out"=w4098:errorcluster, "wait_expose"=w4097:bool, "Channel out"=w4100:refnum<class "Channel.lvclass">)  [unwired: 7 in]
              n1466 = call-dynamic "Read State Machine.vi"("error in (no error)"=w4098, "Device in"=w4100) -> ("error out"=w4106:errorcluster, "State Machine.lvclass"=w4108:refnum<class "State Machine.lvclass">, "Device out"=w4110:refnum<class "Channel.lvclass">)  [unwired: 7 in]
              n1467 = call-dynamic "Read State.vi"("error in (no error)"=w4106, "State Machine in"=w4108) -> ("error out"=w4105:errorcluster, "State"=w4103:i32, "State Machine out"=w4107:refnum<class "State Machine.lvclass">)  [unwired: 7 in]
              n1468 = Greater?(x=w4103, y=53 ("x")) -> (0:w4102:bool)
              n1469 = call-dynamic "Write State Machine.vi"("error in (no error)"=w4105, "State Machine.lvclass"=w4107, "Device in"=w4110) -> ("error out"=w4109:errorcluster, "Device out"=w4111:refnum<class "Channel.lvclass">)  [unwired: 7 in]
              n1470 = call-dynamic "Write Channel.vi"("error in (no error)"=w4109, "Channel.lvclass"=w4111, "Acquisition in"=w4112) -> ("error out"=w4115:errorcluster, "Acquisition out"=w4116:refnum<class "Acquisition.lvclass">)  [unwired: 7 in]
            }
          }
          n1471 = call-dynamic "Write AcquisitionD.vi"("error in (no error)"=w4072, "Acquisition.lvclass"=w4073, "S4ACS_GUI in"=w4071) -> ("error out"=w4063:errorcluster, "S4ACS_GUI out"=w4033:refnum<class "S4GUI.lvclass">)  [unwired: 7 in]
          n1472 = Compound Arithmetic op=AND(w4040, w4042, w4041, w4039) -> (w4032:bool)
          n1473 = Compound Arithmetic op=OR(w4038, w4037, w4036, w4035) -> (w4034:bool)
          n1474 = case shown="False" w4032 {
            tunnel: w4033 -> [w4087 w4092]
            tunnel: [w4088 w4091] -> w4030
            tunnel: w4031 -> [w4086 _]
            frame False {
              n1475 = Increment(x=w4086) -> (x+1=w4085:u32)
              n1476 = Bundle By Name(cluster=w4087, "Obs_state"=w4085) -> (w4088:refnum<class "S4GUI.lvclass">)
            }
            frame True {
              # "ACTIVE detectado.\nIniciou aquisição..."
              n1477 = Tick Count (ms)() -> (millisecond timer value=w4089:u32)
              n1478 = local write "time307"(w4089) -> ()
              n1479 = Bundle By Name(cluster=w4092, "Obs_state"=u32 328) -> (w4091:refnum<class "S4GUI.lvclass">)
            }
          }
          n1480 = Bundle By Name(cluster=w4030, "mode EXPOSE"=w4034) -> (w4079:refnum<class "S4GUI.lvclass">)
        }
        frame 327 {
          # "T= canais receberam STOP"
          n1481 = Unbundle By Name(w4216) -> ("cyclesDone"=w4211:u32)
          n1482 = call-dynamic "Read AcquisitionA.vi"("error in (no error)"=w4249, "S4ACS_GUI in"=w4216) -> ("error out"=w4231:errorcluster, "Acquisition.lvclass"=w4232:refnum<class "Acquisition.lvclass">, "S4ACS_GUI out"=w4251:refnum<class "S4GUI.lvclass">)  [unwired: 7 in]
          n1483 = call-dynamic "Read enabled.vi"("error in (no error)"=w4231, "Server in"=w4232) -> ("error out"=w4230:errorcluster, "enabled"=w4207:bool, "Server out"=w4229:refnum<class "Acquisition.lvclass">)  [unwired: 7 in]
          n1484 = case shown="True" w4207 {
            tunnel: w4230 -> [w4402 w4419]
            tunnel: [w4403 w4417] -> w4252
            tunnel: [w4402 w4416] -> w4250
            tunnel: [0 ("State") w4412] -> w4202
            tunnel: w4229 -> [w4403 w4411]
            tunnel: w4211 -> [_ w4410]
            tunnel: [TRUE w4409] -> w4215
            tunnel: [FALSE ("stopping") w4405] -> w4198
            frame False {
            }
            frame True {
              n1485 = call-dynamic "Read Channel.vi"("error in (no error)"=w4419, "Acquisition in"=w4411) -> ("error out"=w4415:errorcluster, "Channel.lvclass"=w4414:refnum<class "Channel.lvclass">, "Acquisition out"=w4418:refnum<class "Acquisition.lvclass">)  [unwired: 7 in]
              n1486 = call-dynamic "Read CyclesDone.vi"("error in (no error)"=w4415, "Channel in"=w4414) -> ("error out"=w4407:errorcluster, "CyclesDone"=w4412:u32, "Channel out"=w4413:refnum<class "Channel.lvclass">)  [unwired: 7 in]
              n1487 = Increment(x=w4410) -> (x+1=w4404:u32)
              n1488 = Equal?(x=w4412, y=w4404) -> (x = y?=w4409:bool)
              n1489 = call-dynamic "Read stopping.vi"("error in (no error)"=w4407, "Channel in"=w4413) -> ("error out"=w4406:errorcluster, "stopping"=w4405:bool, "Channel out"=w4408:refnum<class "Channel.lvclass">)  [unwired: 7 in]
              n1490 = call-dynamic "Write Channel.vi"("error in (no error)"=w4406, "Channel.lvclass"=w4408, "Acquisition in"=w4418) -> ("error out"=w4416:errorcluster, "Acquisition out"=w4417:refnum<class "Acquisition.lvclass">)  [unwired: 7 in]
            }
          }
          n1491 = call-dynamic "Write AcquisitionA.vi"("error in (no error)"=w4250, "Acquisition.lvclass"=w4252, "S4ACS_GUI in"=w4251) -> ("error out"=w4247:errorcluster, "S4ACS_GUI out"=w4246:refnum<class "S4GUI.lvclass">)  [unwired: 7 in]
          n1492 = call "Read AcquisitionB.vi"("error in (no error)"=w4247, "S4ACS_GUI in"=w4246) -> ("error out"=w4225:errorcluster, "Acquisition.lvclass"=w4228:refnum<class "Acquisition.lvclass">, "S4ACS_GUI out"=w4248:refnum<class "S4GUI.lvclass">)  [unwired: 7 in]
          n1493 = call-dynamic "Read enabled.vi"("error in (no error)"=w4225, "Server in"=w4228) -> ("error out"=w4226:errorcluster, "enabled"=w4206:bool, "Server out"=w4227:refnum<class "Acquisition.lvclass">)  [unwired: 7 in]
          n1494 = case shown="True" w4206 {
            tunnel: w4226 -> [w4381 w4398]
            tunnel: w4227 -> [w4382 w4397]
            tunnel: [0 ("State") w4390] -> w4201
            tunnel: [w4381 w4396] -> w4245
            tunnel: [w4382 w4395] -> w4244
            tunnel: w4211 -> [_ w4389]
            tunnel: [TRUE w4388] -> w4212
            tunnel: [FALSE ("stopping") w4384] -> w4197
            frame False {
            }
            frame True {
              n1495 = call-dynamic "Read Channel.vi"("error in (no error)"=w4398, "Acquisition in"=w4397) -> ("error out"=w4393:errorcluster, "Channel.lvclass"=w4394:refnum<class "Channel.lvclass">, "Acquisition out"=w4391:refnum<class "Acquisition.lvclass">)  [unwired: 7 in]
              n1496 = call-dynamic "Read CyclesDone.vi"("error in (no error)"=w4393, "Channel in"=w4394) -> ("error out"=w4386:errorcluster, "CyclesDone"=w4390:u32, "Channel out"=w4392:refnum<class "Channel.lvclass">)  [unwired: 7 in]
              n1497 = Increment(x=w4389) -> (x+1=w4383:u32)
              n1498 = Equal?(x=w4390, y=w4383) -> (x = y?=w4388:bool)
              n1499 = call-dynamic "Read stopping.vi"("error in (no error)"=w4386, "Channel in"=w4392) -> ("error out"=w4385:errorcluster, "stopping"=w4384:bool, "Channel out"=w4387:refnum<class "Channel.lvclass">)  [unwired: 7 in]
              n1500 = call-dynamic "Write Channel.vi"("error in (no error)"=w4385, "Channel.lvclass"=w4387, "Acquisition in"=w4391) -> ("error out"=w4396:errorcluster, "Acquisition out"=w4395:refnum<class "Acquisition.lvclass">)  [unwired: 7 in]
            }
          }
          n1501 = Max & Min(x=w4202, y=w4201) -> (max(x,y)=w4214:u32)  [unwired: 1 out]
          n1502 = call "Write AcquisitionB.vi"("error in (no error)"=w4245, "Acquisition.lvclass"=w4244, "S4ACS_GUI in"=w4248) -> ("error out"=w4237:errorcluster, "S4ACS_GUI out"=w4236:refnum<class "S4GUI.lvclass">)  [unwired: 7 in]
          n1503 = call-dynamic "Read AcquisitionC.vi"("error in (no error)"=w4237, "S4ACS_GUI in"=w4236) -> ("error out"=w4222:errorcluster, "Acquisition.lvclass"=w4224:refnum<class "Acquisition.lvclass">, "S4ACS_GUI out"=w4239:refnum<class "S4GUI.lvclass">)  [unwired: 7 in]
          n1504 = call-dynamic "Read enabled.vi"("error in (no error)"=w4222, "Server in"=w4224) -> ("error out"=w4221:errorcluster, "enabled"=w4205:bool, "Server out"=w4223:refnum<class "Acquisition.lvclass">)  [unwired: 7 in]
          n1505 = case shown="True" w4205 {
            tunnel: [w4360 w4377] -> w4240
            tunnel: [w4361 w4376] -> w4238
            tunnel: w4221 -> [w4360 w4373]
            tunnel: w4223 -> [w4361 w4374]
            tunnel: [0 ("State") w4372] -> w4200
            tunnel: w4211 -> [_ w4371]
            tunnel: [TRUE w4370] -> w4210
            tunnel: [FALSE ("stopping") w4363] -> w4196
            frame False {
            }
            frame True {
              n1506 = call-dynamic "Read Channel.vi"("error in (no error)"=w4373, "Acquisition in"=w4374) -> ("error out"=w4369:errorcluster, "Channel.lvclass"=w4368:refnum<class "Channel.lvclass">, "Acquisition out"=w4375:refnum<class "Acquisition.lvclass">)  [unwired: 7 in]
              n1507 = call-dynamic "Read CyclesDone.vi"("error in (no error)"=w4369, "Channel in"=w4368) -> ("error out"=w4365:errorcluster, "CyclesDone"=w4372:u32, "Channel out"=w4367:refnum<class "Channel.lvclass">)  [unwired: 7 in]
              n1508 = Increment(x=w4371) -> (x+1=w4362:u32)
